vi "workbook.free.vi"(8 "error in":errorcluster, 11 "Workbook":refnum<class "Workbook.lvclass">) -> (0 "error out":errorcluster)   [LabVIEW 2020, in "Workbook.lvclass"]
doc: "Releases the handle and its associated resources."
uses:
  Workbook.lvclass
  Workbook.lvclass/Workbook.ctl
  client.lvlib
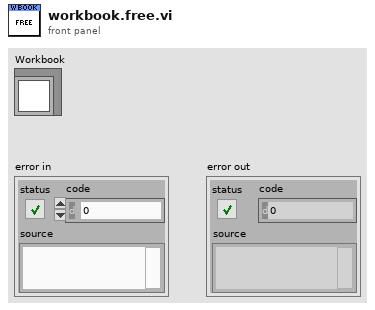
[diagram p1: front panel]
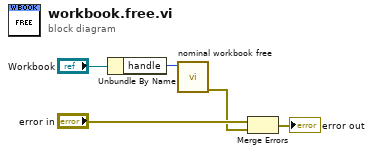
[diagram p0: block diagram]
diagram:
  n1 = Unbundle By Name("Workbook") -> ("handle"=w5:i32)
  n2 = call "nominal workbook free.vi"("workbook"=w5) -> ("error out"=w2:errorcluster)  [unwired: 9 in, 1 out]
  n3 = Merge Errors("error in", w2) -> (→"error out":errorcluster)
